vi "Get Control Refnum and Tab by Name.vi"(8 "error in":errorcluster, 9 "Selection":T1(ring), 10 "Control Label":string, 11 "VI  Ref":refnum<vi>) -> (0 "error out":errorcluster, 1 "Owning Tab Name":string, 2 "Ctl Refnum":refnum<vi>, 3 "VI  Ref (dup)":refnum<vi>, 4 "Ctl found?":bool)   [LabVIEW 2021]
doc: "Returns an array of control refnums, labels and data, from the front panel of the calling VI.\n\nThis VI also accounts for tab controls within other tab controls."
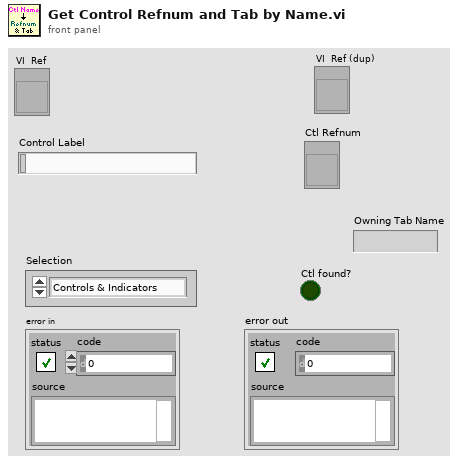
[diagram p1: front panel]
types:
  T1 = enum16{"Controls & Indicators", "Controls", "Indicators"}
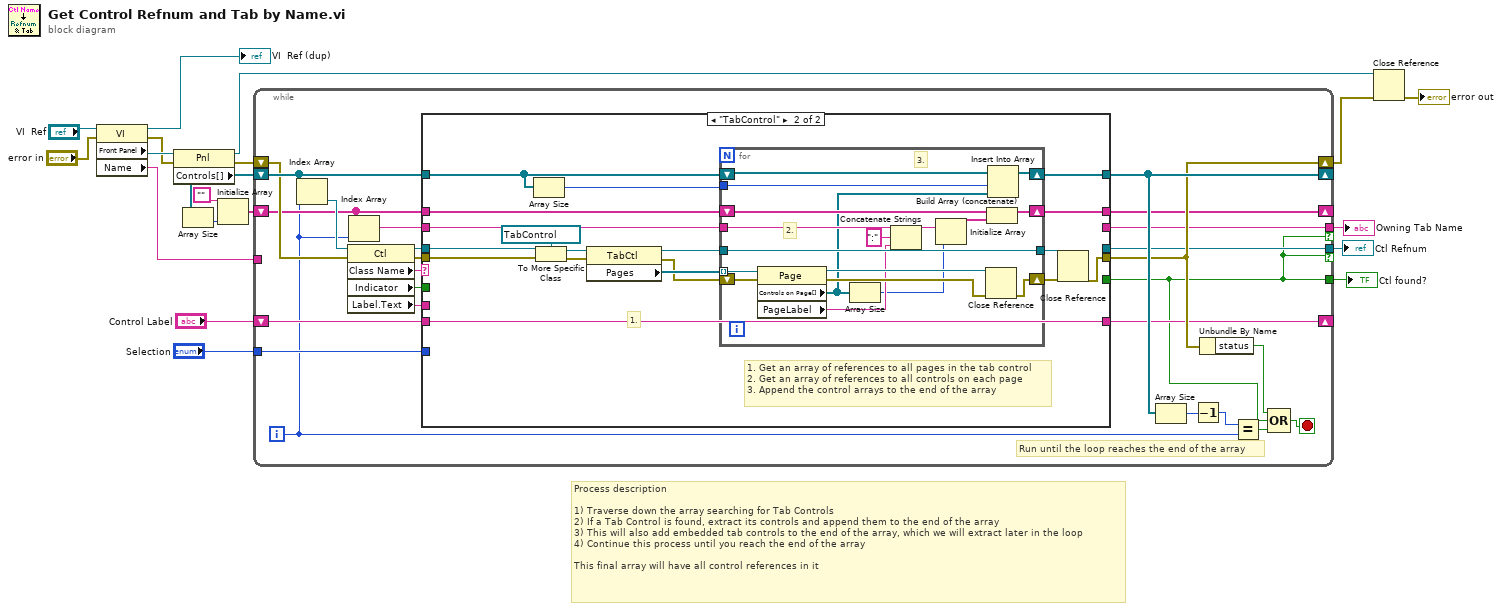
[diagram p0: block diagram]
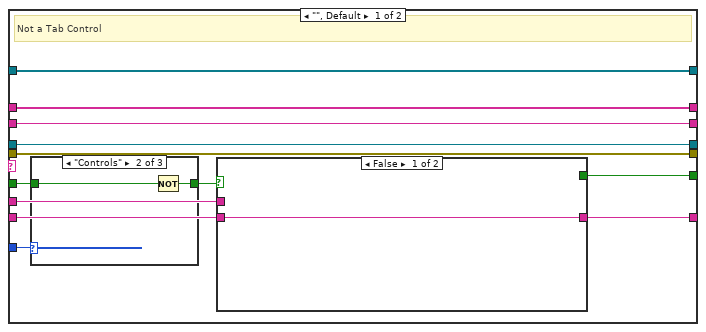
[diagram p2: hidden frame]
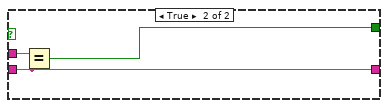
[diagram p3: hidden frame]
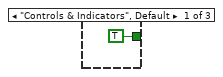
[diagram p4: hidden frame]
diagram:
  # "Process description\n\n1) Traverse down the array searching for Tab Controls\n2) If a Tab Control is found, extract its controls and append them to the end of the array\n3) This will also add embedded tab controls to the end of the array, which we will extract later in the loop\n4) Continue this process until you reach the end of the array\n\nThis final array will have all control references in it"
  n1 = property class="VI"(reference="VI  Ref", error in="error in") -> (reference out=→"VI  Ref (dup)":refnum<vi>, error out=w18:errorcluster, "Front Panel"=w19:refnum<vi>, "Name"=w1:string)
  n2 = property class="Pnl"(reference=w19, error in=w18) -> (reference out=w16:refnum<vi>, error out=w17:errorcluster, "Controls[]"=w6:refnum<vi>[])
  n3 = Array Size(array=w6) -> (size(s)=w5:i32)
  n4 = Initialize Array("", w5) -> (w3:string[])
  n5 = while {
    shift-right: [w38] -> _
    shift-left: w6 -> [w43]
    shift-right: [w35] -> w15
    shift-left: w17 -> [w37]
    shift-right: [w28] -> _
    shift-left: "Control Label" -> [w30]
    tunnel: [w29] -> w9 if=w20
    tunnel: "Selection" -> [w26]
    tunnel: [w20] -> w7
    shift-right: [w25] -> _
    shift-left: w3 -> [w24]
    tunnel: [w21] -> w2 if=w20
    tunnel: w1 -> [_]
    i -> [w23]
    stop <- w33 stop-if-true
    # "Run until the loop reaches the end of the array"
    n6 = Index Array(array=w43, index=w23) -> (element=w39:refnum<vi>)
    n7 = property class="Ctl"(reference=w39, error in=w37) -> (reference out=w44:refnum<vi>, error out=w36:errorcluster, "Class Name"=w42:string, "Indicator"=w27:bool, "Label.Text"=w31:string)
    n8 = Index Array(array=w24, index=w23) -> (element=w22:string)
    n9 = case shown="\"TabControl\"" w42 {
      tunnel: w44 -> [w53 w82]
      tunnel: w43 -> [w56 w78]
      tunnel: [w56 w79] -> w38
      tunnel: w36 -> [w55 w75]
      tunnel: [w55 w71] -> w35
      tunnel: w31 -> [w54 _]
      tunnel: w30 -> [w51 w68]
      tunnel: [w53 _] -> w29
      tunnel: [w52 _] -> w20
      tunnel: [w50 w68] -> w28
      tunnel: w27 -> [w48 _]
      tunnel: w26 -> [w49 _]
      tunnel: w24 -> [w46 w67]
      tunnel: [w46 w66] -> w25
      tunnel: w22 -> [w45 w65]
      tunnel: [w45 _] -> w21
      frame "", Default {
        # "Not a Tab Control"
        n10 = case shown="\"Controls\"" w49 {
          tunnel: w48 -> [_ w63 w64]
          tunnel: [TRUE ("Indicator") w62 w64] -> w47
          frame "Controls & Indicators", Default {
          }
          frame "Controls" {
            n11 = Not(x=w63) -> (.not. x?=w62:bool)
          }
          frame "Indicators" {
          }
        }
        n12 = case shown="False" w47 {
          tunnel: w54 -> [_ w59]
          tunnel: [_ w58] -> w52
          tunnel: w51 -> [w57 w60]
          tunnel: [w57 w60] -> w50
          frame False {
          }
          frame True {
            n13 = Equal?(x=w59, y=w60) -> (x = y?=w58:bool)
          }
        }
      }
      frame "TabControl" {
        # "1. Get an array of references to all pages in the tab control\n2. Get an array of references to all controls on each page\n3. Append the control arrays to the end of the array"
        # "1."
        n14 = Array Size(array=w78) -> (size(s)=w76:i32)
        n15 = To More Specific Class(target class=refnum<vi> refnum ("Tab Control"), reference=w82, error in=w75) -> (specific class reference=w81:refnum<vi>, error out=w74:errorcluster)
        n16 = property class="TabCtl"(reference=w81, error in=w74) -> (reference out=w72:refnum<vi>, error out=w73:errorcluster, "Pages"=w80:refnum<vi>[])
        n17 = for {
          tunnel: w80 -> [w100] mode=indexing
          tunnel: w76 -> [w98]
          shift-right: [w99] -> w79
          shift-left: w78 -> [w97]
          tunnel: w72 -> [w95]
          tunnel: [w95] -> w70
          shift-right: [w92] -> w69
          shift-left: w73 -> [w96]
          shift-right: [w90] -> w66
          shift-left: w67 -> [w91]
          tunnel: w65 -> [w89]
          # "3."
          # "2."
          n18 = property class="Page"(reference=w100, error in=w96) -> (reference out=w94:refnum<vi>, error out=w93:errorcluster, "Controls on Page[]"=w85:refnum<vi>[], "PageLabel"=w87:string)
          n19 = Array Size(array=w85) -> (size(s)=w84:i32)
          n20 = Concatenate Strings(w89, ":" ("string"), w87) -> (w86:string)
          n21 = Initialize Array(w86, w84) -> (w83:string[])
          n22 = Close Reference(reference=w94, error in (no error)=w93) -> (error out=w92:errorcluster)
          n23 = Build Array (concatenate)(w91, w83) -> (w90:string[])
          n24 = Insert Into Array(array=w97, index=w98, new element=w85) -> (w99:refnum<vi>[])
        }
        n25 = Close Reference(reference=w70, error in (no error)=w69) -> (error out=w71:errorcluster)
      }
    }
    n26 = Array Size(array=w38) -> (size(s)=w41:i32)
    n27 = Decrement(x=w41) -> (x-1=w40:i32)
    n28 = Unbundle By Name(w35) -> ("status"=w32:bool)
    n29 = Equal?(x=w40, y=w23) -> (x = y?=w34:bool)
    n30 = Compound Arithmetic op=OR(w32, w20, w34) -> (w33:bool)
  }
  "Ctl found?" <- w7
  "Ctl Refnum" <- w9
  "Owning Tab Name" <- w2
  n31 = Close Reference(reference=w16, error in (no error)=w15) -> (error out=→"error out":errorcluster)
